vi "选择图片.vi"() -> (3 "图像路径 2":path)   [LabVIEW 2018]
panel:
  in  "打开图像":bool
  in  "图像路径":path
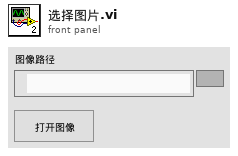
[diagram p1: front panel]
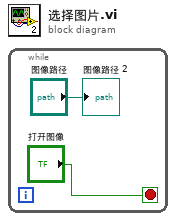
[diagram p0: block diagram]
diagram:
  n1 = while {
    stop <- "打开图像" stop-if-true
    "图像路径 2" <- "图像路径"
  }
